vi "sub_WriteConfiguration.vi"(6 "create file if necessary? (T)":bool=TRUE caption="必要时创建文件？(T)", 8 "error in (no error)":errorcluster, 10 "INI Fomatted Cluster":variant, 11 "configuration file path":path caption="配置文件的路径") -> (0 "error out":errorcluster)   [LabVIEW 2013, in "0_SystemCOnfiguration.lvlib"]
uses:
  0_SystemCOnfiguration.lvlib
  <vilib>/Utility/config.llb/NI_LVConfig.lvlib
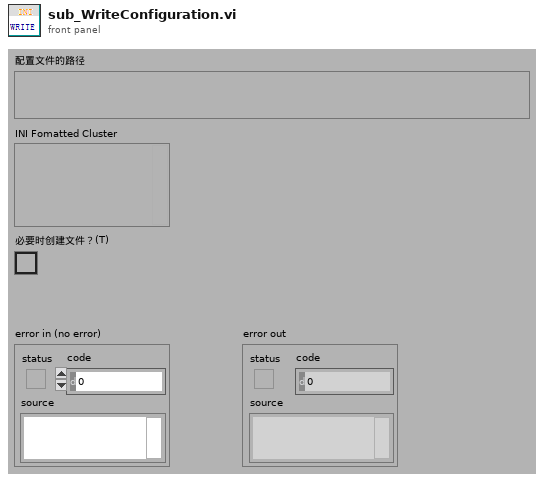
[diagram p1: front panel]
types:
  T1 = typedef "NI_LVConfig.lvlib/Config Data RefNum.ctl" = refnum<k1>
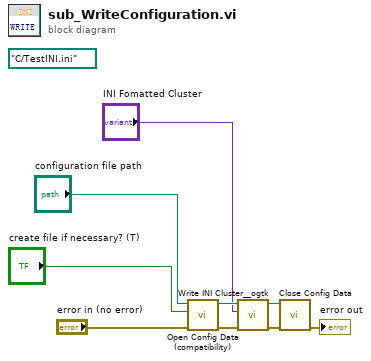
[diagram p0: block diagram]
diagram:
  (unwired) path "C:/TestINI.ini" ("configuration file path")
  n1 = call <vilib>:"Open Config Data (compatibility).vi"("error in (no error)"="error in (no error)", "create file if necessary (T)"="create file if necessary? (T)", "configuration file path"="configuration file path") -> ("error out"=w9:errorcluster, "refnum"=w8:T1)  [unwired: 6 in, 1 out]
  n2 = call <userlib>:"Write INI Cluster__ogtk.vi"("error in (no error)"=w9, "INI Fomatted Cluster"="INI Fomatted Cluster", "refnum"=w8) -> ("error out"=w6:errorcluster, "dup refnum"=w7:T1)  [unwired: 7 in]
  n3 = call <vilib>:"Close Config Data.vi"("error in (no error)"=w6, "refnum"=w7) -> ("error out"=→"error out":errorcluster)  [unwired: 8 in, 1 out]
